vi "DCA Convert 1.9 to 1.10 - 1.11.vi"(0 "DCA 1.9 Test Parameters":T12={"Stimulus"={"Use Instrument"=FALSE, "Normalize"=FALSE, "Blank Screen"=FALSE, "Measurement Type"=enum."Voltage DC", "Range"=enum."Auto", "Resolution"=enum."Auto"}, "Measurement"={"Topology"=enum."PI-Network", "Lock Topology"=FALSE, "ATTN Calc"=enum."Power", "Zo"=50.0}, "Limits"=[], "Datasheets"=[]}) -> (1 "Datasheets":T1, 2 "DCA 1.10 - 1.11 Test Parameters":T2={"Stimulus"={"Use Instrument"=FALSE, "Normalize"=FALSE, "Blank Screen"=FALSE, "Measurement Type"=enum."Diode", "Range"=enum."Auto", "Resolution"=enum."Auto"}, "Measurement"={"Topology"=enum."PI-Network", "Lock Topology"=FALSE, "ATTN Calc"=enum."Power", "Zo"=50.0}, "Limits"=[]})   [LabVIEW 2011]
uses:
  TypeDefs/DCA Test Parameters v1.9.ctl
  TypeDefs/DCA Test Parameters v1.10-1.11.ctl
  TypeDefs/DCA Stimulus Parameters.ctl
  TypeDefs/DCA Measurement Cluster.ctl
  TypeDefs/DCA Topology.ctl
  TypeDefs/DCA Attenuation Calculation.ctl
  TypeDefs/DCA Limit.ctl
  TypeDefs/DCA Limit Quantity.ctl
  TypeDefs/DCA Limit Comparison.ctl
  TypeDefs/DCA Limit Operation.ctl
  Test Referential Limit.ctl
  Test Datasheets v1.0-4.0.ctl
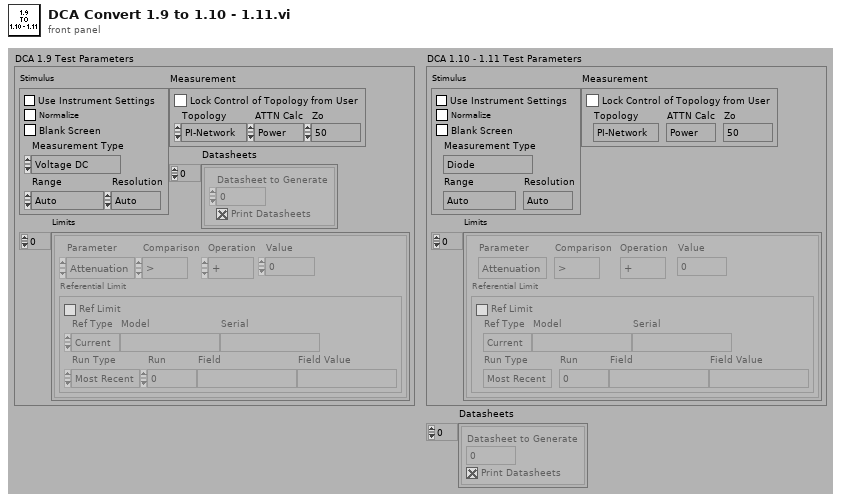
[diagram p1: front panel]
types:
  T1 = typedef "Test Datasheets v1.0-4.0.ctl" = cluster{"Datasheet to Generate":i32, "Print Datasheets":bool}[]
  T2 = typedef "DCA Test Parameters v1.10-1.11.ctl" = cluster{"Stimulus":T3, "Measurement":T4, "Limits":T7[]}
  T3 = typedef "DCA Stimulus Parameters.ctl" = cluster{"Use Instrument":bool, "Normalize":bool, "Blank Screen":bool, "Measurement Type":enum16{"Voltage DC", "Voltage DC Ratio", "Voltage AC", "Current DC", "Current AC", "Resistance", "Fresistance", "Frequency", "Period", "Continuity", "Diode"}, "Range":enum16{"Auto", "Minimum", "Maximum", "100", "1,000", "10,000", "100,000", "1,000,000", "10,000,000", "100,000,000"}, "Resolution":enum16{"Auto", "4 1/2", "5 1/2", "6 1/2"}}
  T4 = typedef "DCA Measurement Cluster.ctl" = cluster{"Topology":T5, "Lock Topology":bool, "ATTN Calc":T6, "Zo":dbl}
  T5 = typedef "DCA Topology.ctl" = enum32{"PI-Network", "T-Network"}
  T6 = typedef "DCA Attenuation Calculation.ctl" = enum32{"Power", "Voltage"}
  T7 = typedef "DCA Limit.ctl" = cluster{"Parameter":T8, "Comparison":T9, "Operation":T10, "Value":dbl, "Referential Limit":T11}
  T8 = typedef "DCA Limit Quantity.ctl" = enum16{"Attenuation", "Zin", "Zout", "R1", "R2", "R3", "Rab", "Rac", "Rbc"}
  T9 = typedef "DCA Limit Comparison.ctl" = enum16{">", ">=", "<", "<="}
  T10 = typedef "DCA Limit Operation.ctl" = enum16{"+", "-"}
  T11 = typedef "Test Referential Limit.ctl" = cluster{"Ref Limit":bool, "Ref Type":enum16{"Current", "Specify"}, "Model":string, "Serial":string, "Run Type":enum16{"Most Recent", "Run #", "Match Field"}, "Run":i32, "Field":string, "Field Value":string}
  T12 = typedef "DCA Test Parameters v1.9.ctl" = cluster{"Stimulus":cluster{"Use Instrument":bool, "Normalize":bool, "Blank Screen":bool, "Measurement Type":enum16{"Voltage DC", "Voltage DC Ratio", "Voltage AC", "Current DC", "Current AC", "Resistance", "Fresistance", "Frequency", "Period", "Continuity", "Diode"}, "Range":enum16{"Auto", "Minimum", "Maximum", "100", "1,000", "10,000", "100,000", "1,000,000", "10,000,000", "100,000,000"}, "Resolution":enum16{"Auto", "4 1/2", "5 1/2", "6 1/2"}}, "Measurement":cluster{"Topology":enum32{"PI-Network", "T-Network"}, "Lock Topology":bool, "ATTN Calc":enum32{"Power", "Voltage"}, "Zo":dbl}, "Limits":cluster{"Parameter":enum16{"Attenuation", "Zin", "Zout", "R1", "R2", "R3", "Rab", "Rac", "Rbc"}, "Comparison":enum16{">", ">=", "<", "<="}, "Operation":enum16{"+", "-"}, "Value":dbl, "Referential Limit":cluster{"Ref Limit":bool, "Ref Type":enum16{"Current", "Specify"}, "Model":string, "Serial":string, "Run Type":enum16{"Most Recent", "Run #", "Match Field"}, "Run":i32, "Field":string, "Field Value":string}}[], "Datasheets":cluster{"Datasheet to Generate":i32, "Print Datasheets":bool}[]}
  T13 = cluster{"Use Instrument":bool, "Normalize":bool, "Blank Screen":bool, "Measurement Type":enum16{"Voltage DC", "Voltage DC Ratio", "Voltage AC", "Current DC", "Current AC", "Resistance", "Fresistance", "Frequency", "Period", "Continuity", "Diode"}, "Range":enum16{"Auto", "Minimum", "Maximum", "100", "1,000", "10,000", "100,000", "1,000,000", "10,000,000", "100,000,000"}, "Resolution":enum16{"Auto", "4 1/2", "5 1/2", "6 1/2"}}
  T14 = cluster{"Topology":enum32{"PI-Network", "T-Network"}, "Lock Topology":bool, "ATTN Calc":enum32{"Power", "Voltage"}, "Zo":dbl}
  T15 = cluster{"Parameter":enum16{"Attenuation", "Zin", "Zout", "R1", "R2", "R3", "Rab", "Rac", "Rbc"}, "Comparison":enum16{">", ">=", "<", "<="}, "Operation":enum16{"+", "-"}, "Value":dbl, "Referential Limit":cluster{"Ref Limit":bool, "Ref Type":enum16{"Current", "Specify"}, "Model":string, "Serial":string, "Run Type":enum16{"Most Recent", "Run #", "Match Field"}, "Run":i32, "Field":string, "Field Value":string}}[]
  T16 = cluster{"Datasheet to Generate":i32, "Print Datasheets":bool}[]
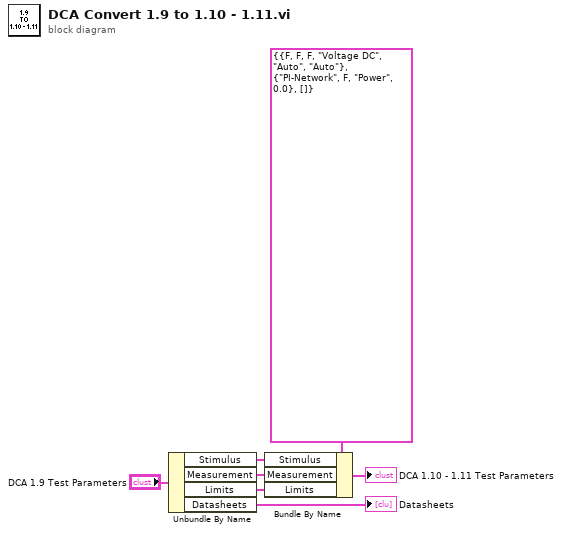
[diagram p0: block diagram]
diagram:
  n1 = Unbundle By Name("DCA 1.9 Test Parameters") -> ("Stimulus"=w5:T13, "Measurement"=w2:T14, "Limits"=w4:T15, "Datasheets"=→"Datasheets":T16)
  n2 = Bundle By Name(cluster=T2 {"Stimulus"={"Use Instrument"=FALSE, "Normalize"=FALSE, "Blank Screen"=FALSE, "Measurement Type"=enum."Voltage DC", "Range"=enum."Auto", "Resolution"=enum."Auto"}, "Measurement"={"Topology"=enum."PI-Network", "Lock Topology"=FALSE, "ATTN Calc"=enum."Power", "Zo"=0.0}, "Limits"=[]} ("DCA 1.9 Test Parameters"), "Stimulus"=w5, "Measurement"=w2, "Limits"=w4) -> (→"DCA 1.10 - 1.11 Test Parameters":T2)
